vi "VLT.vi"() -> ()   [LabVIEW 2025]
uses:
  <vilib>/sound2/lvsound2.llb/Sound Data Format.ctl
  <vilib>/sound2/lvsound2.llb/Sampling Mode.ctl
  <vilib>/sound2/lvsound2.llb/Sound Input Task ID.ctl
  <vilib>/sound2/lvsound2.llb/Sound Output Task ID.ctl
  <vilib>/sound2/lvsound2.llb/Sound Output Write (DBL Single).vi
  <vilib>/sound2/lvsound2.llb/Sound Output Set Volume (Single).vi
  <vilib>/sound2/lvsound2.llb/Sound Input Read (DBL).vi
  <vilib>/Analysis/NI_AALBase.lvlib
  <vilib>/measure/NI_MABase.lvlib
  <vilib>/Utility/inputDevices.llb/joystickAcquire.vi
  <vilib>/sound2/lvsound2.llb/Sound Output Write (DBL).vi
  <vilib>/sound2/lvsound2.llb/Sound File Write Open.vi
  <vilib>/sound2/lvsound2.llb/Sound File Write (DBL).vi
panel:
  in  "Tone Volume":dbl(slide) scale=0.0..1.0 scale format="%_1f"
  out "sample rate (S/s)":dbl
  in  "Sound Waves 2":u16(ring) items=["Sine Wave", "Triangle Wave", "Sawtooth Wave"]
  out "Tone Generator 2":dbl
  out "Number of Samples/ch":i32=20000
  in  "Exit":bool
  in  "stapu 2":bool
  in  "Stop Program":bool
  in  "Input Devicea ID":dbl
  in  "Output Volume":dbl(slide) scale=0.0..100.0
  in  "Sound Devicea ID":dbl
  in  "Pause":bool
  out "Error Write":bool
  in  "Sound Format":T1={"sample rate (S/s)"=22050.0, "number of channels"=2, "bits per sample"=16}
  in  "Record Stop":bool
  out "Error Read":bool
  in  "VLT":T2(tab)
  in  "Playback":bool
  out "Pitch (Hz)":dbl format="%#.2f"
  out "Amplitude Tracker":dynamicdata(graph) caption="Frequency"
  out "Pitch Tracker":waveform(dbl)(graph) caption="Frequency"
  out "Low (Hz)":dbl format="%#.1f"
  out "High (Hz)":dbl format="%#.1f"
  out "Volume (dB)":dbl format="%#.2f"
  out "High (dB)":dbl format="%#.2f"
  out "Low (dB)":dbl format="%#.2f"
  in  "Sound Patterns":u16(ring)
  in  "Sound Waves":u16(ring) items=["Sine Wave", "Triangle Wave", "Sawtooth Wave", "Test"]
  in  "Tone Buttons":T3(radio)=enum."92"
  out "Sound Input":dbl format="%#.0f"
  out "Tone Generator":u32
  # "Hz"
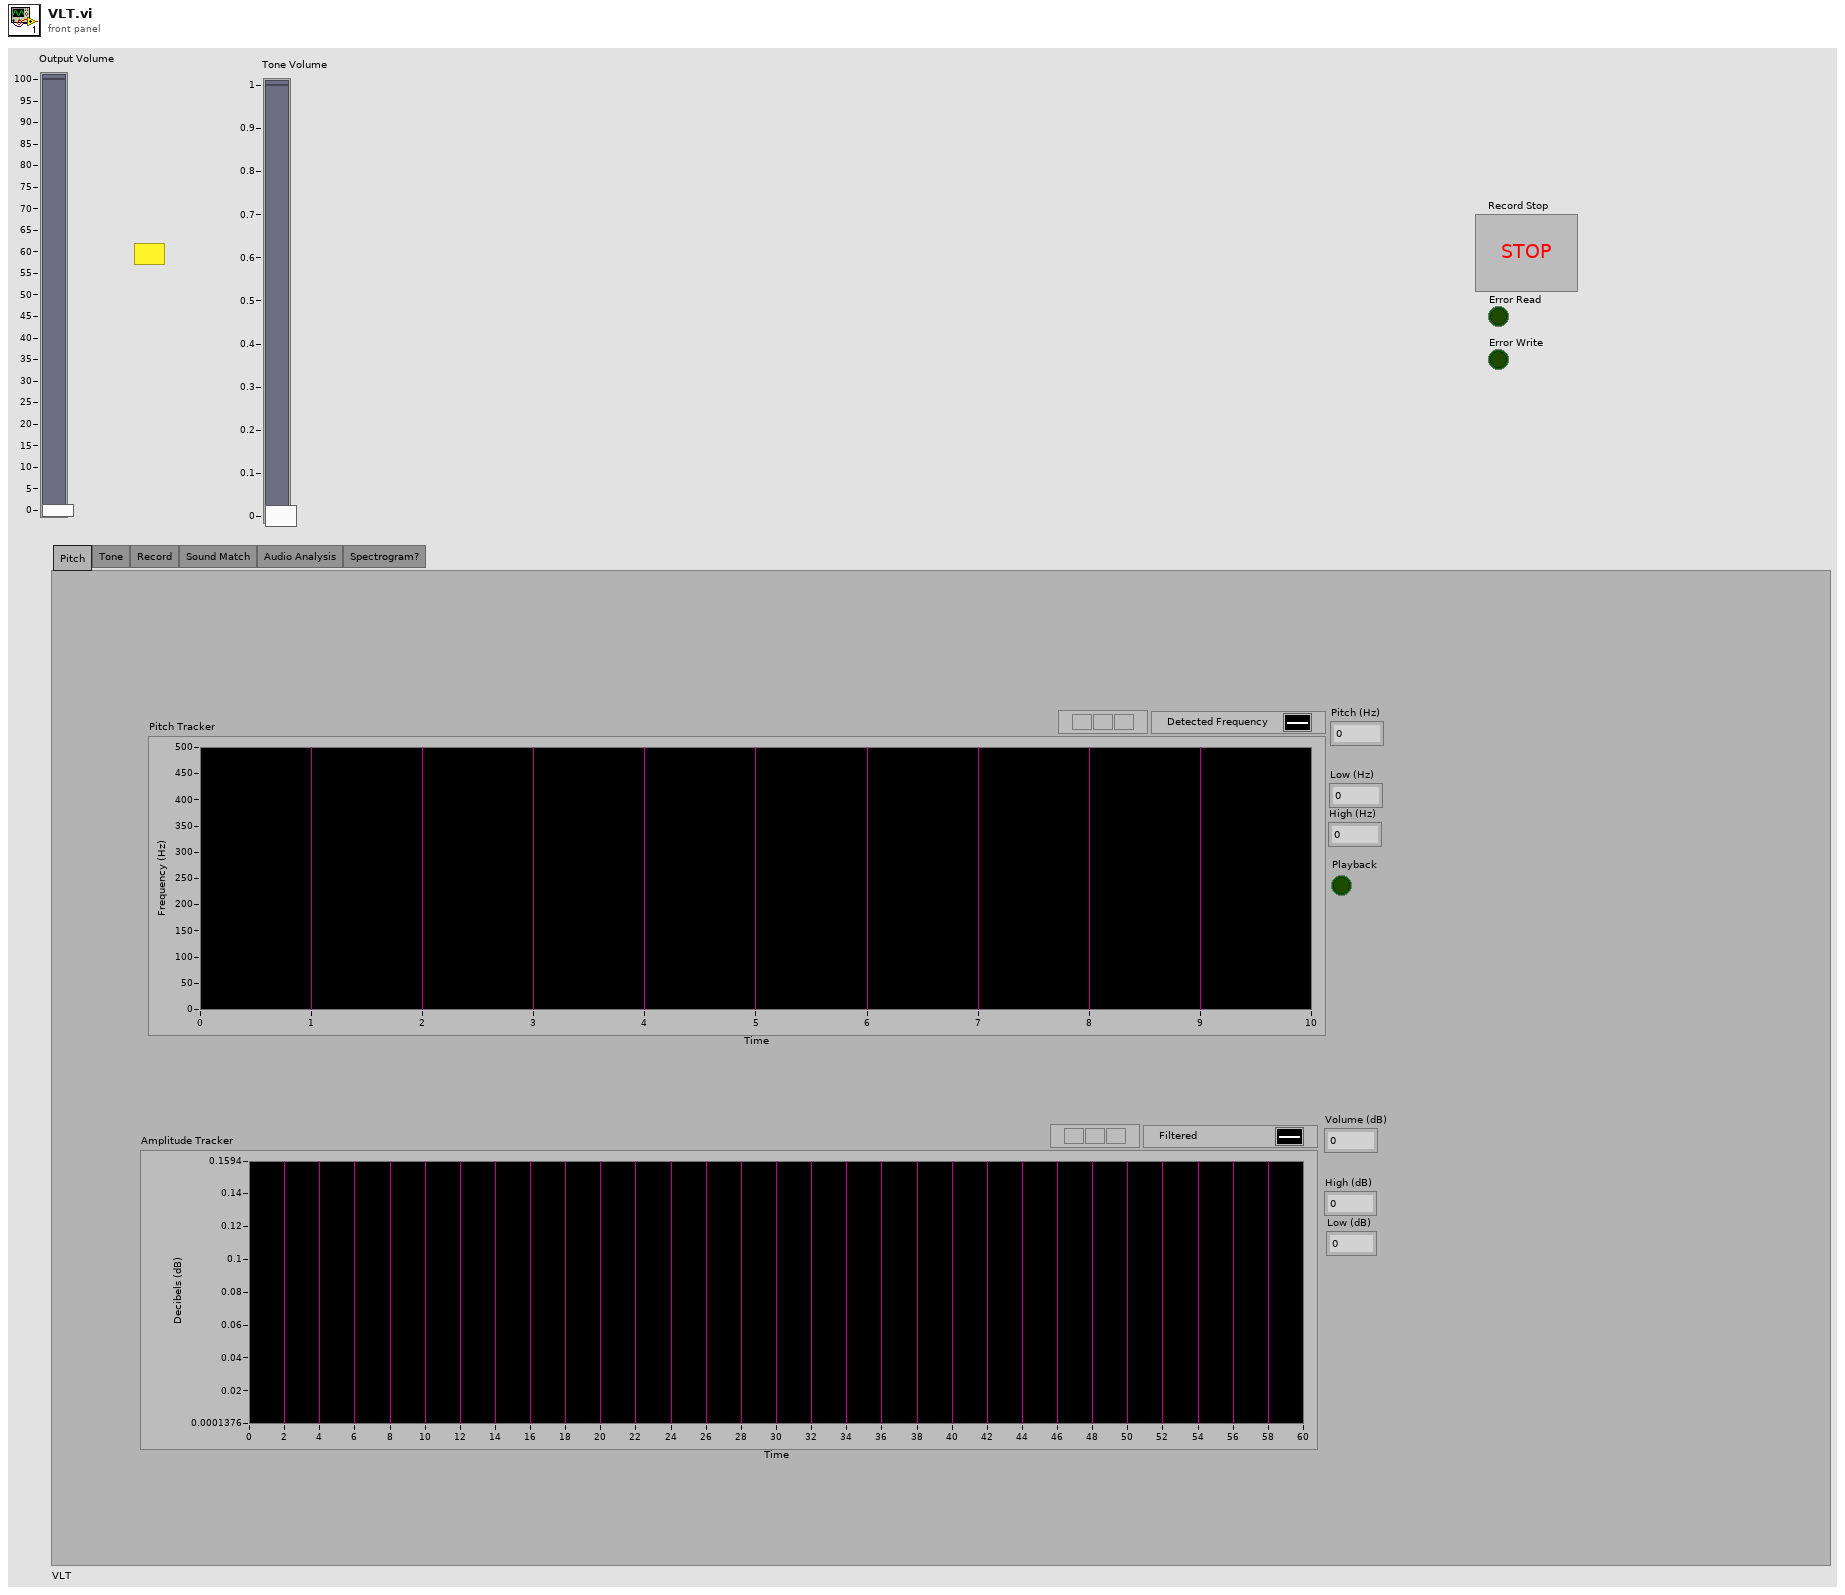
[diagram p1: front panel]
types:
  T1 = typedef "Sound Data Format.ctl" = cluster{"sample rate (S/s)":dbl, "number of channels":i32, "bits per sample":i32}
  T2 = enum32{"Pitch", "Tone", "Record", "Sound Match", "Audio Analysis", "Spectrogram?"}
  T3 = enum32{"No Selection", "92", "98", "104", "110", "117", "123", "175", "165", "156", "131", "139", "147", "247", "233", "220", "185", "196", "208", "349", "330", "311", "262", "277", "294"}
  T4 = typedef "Sound Output Task ID.ctl" = u32
  T5 = typedef "Sound Input Task ID.ctl" = u32
  T6 = typedef "Sampling Mode.ctl" = i32
  T7 = typedef "Sound File Refnum.ctl" = refnum<file>
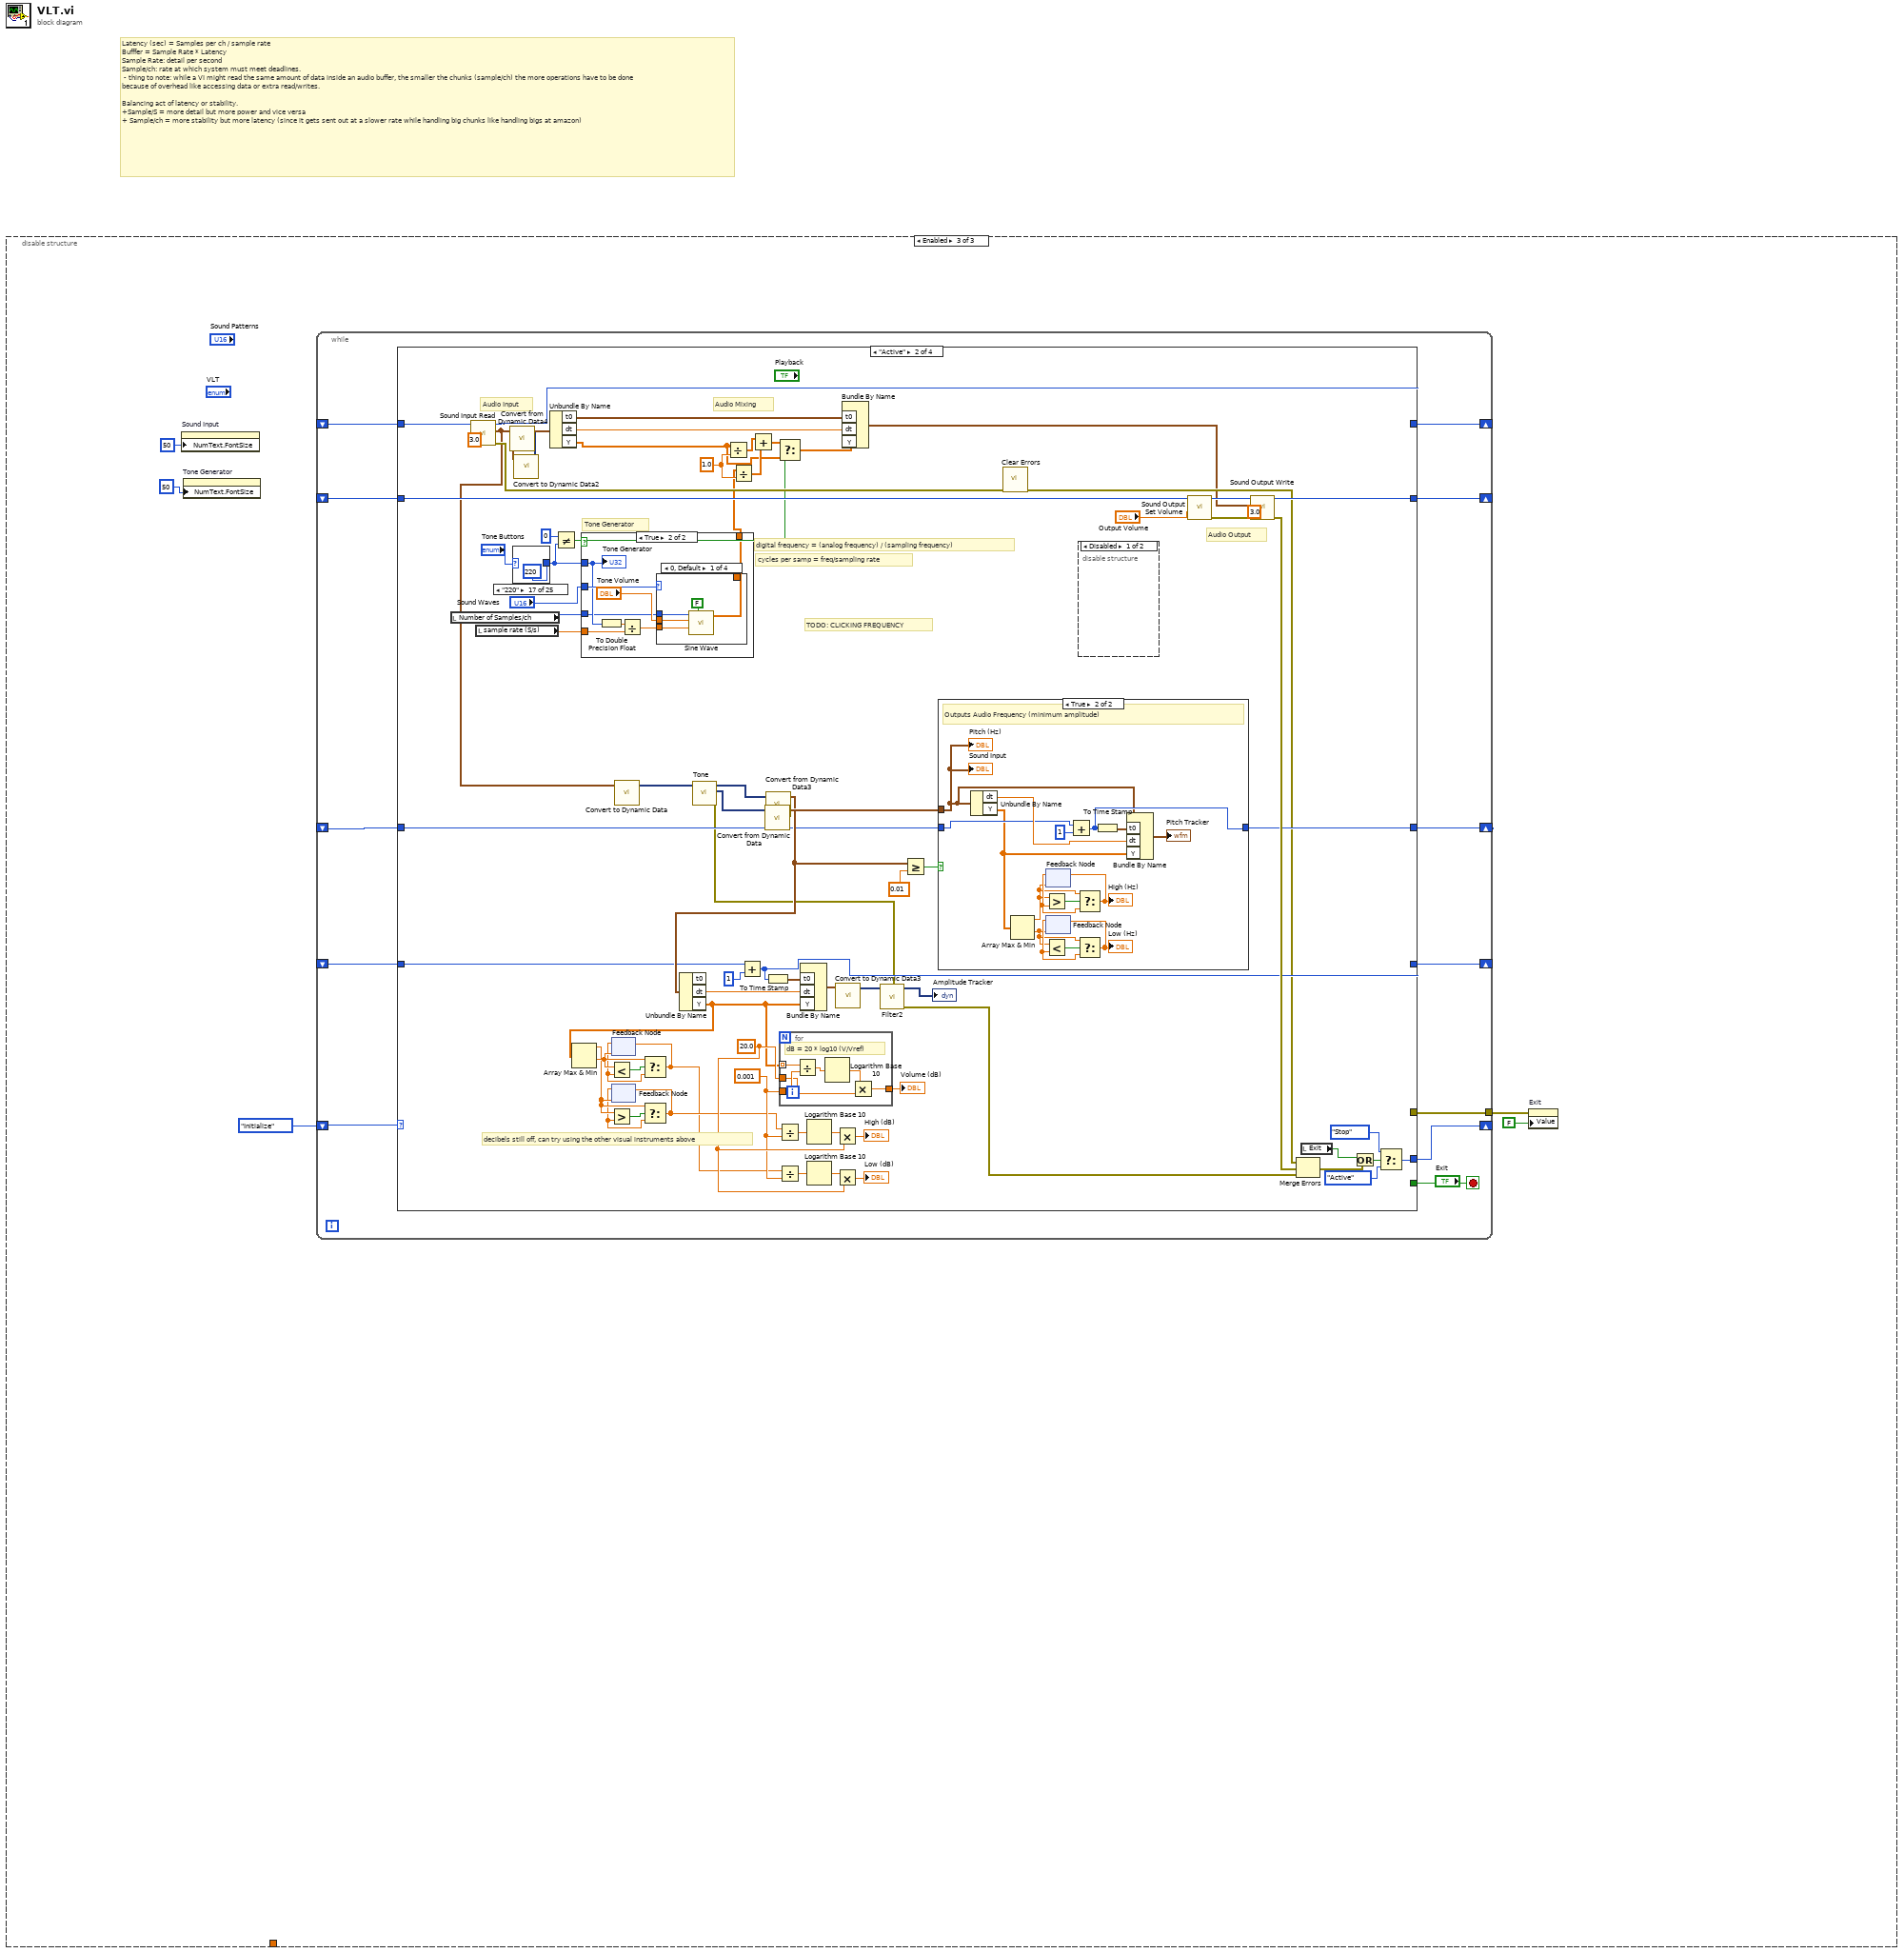
[diagram p0: block diagram]
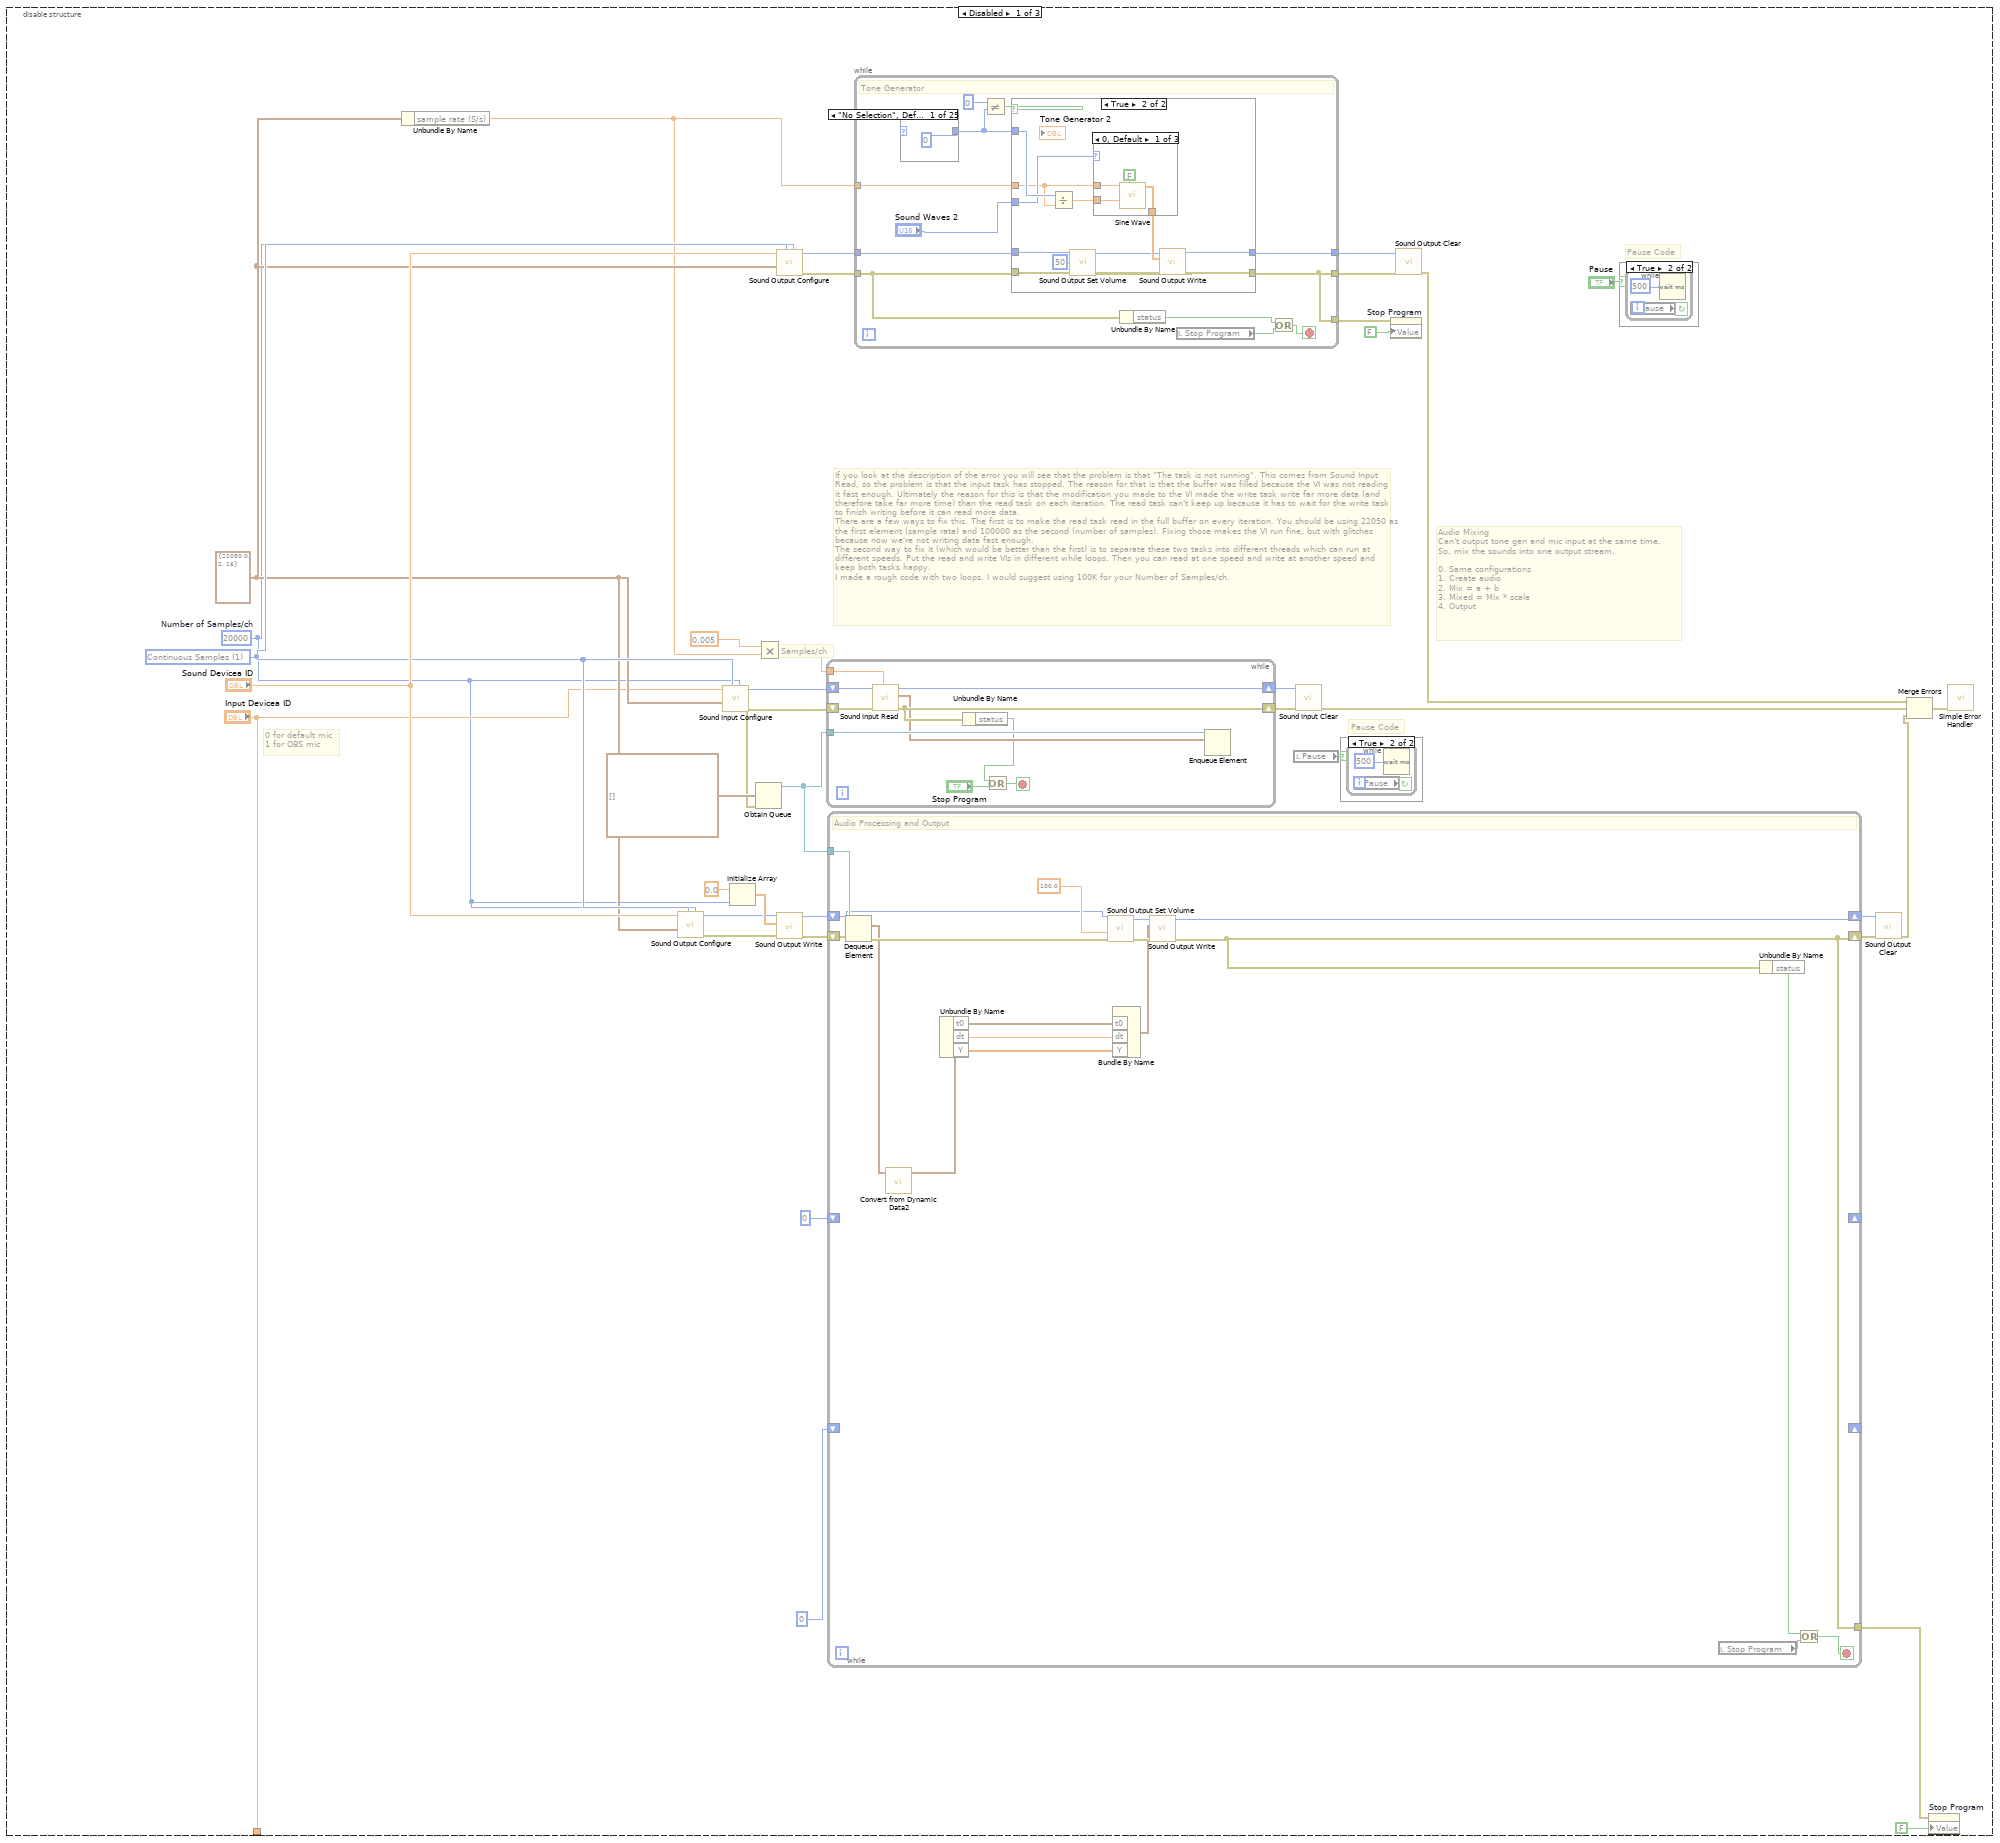
[diagram p2: hidden frame]
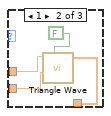
[diagram p6: hidden frame]
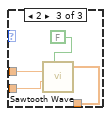
[diagram p7: hidden frame]
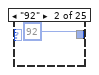
[diagram p8: hidden frame]
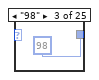
[diagram p9: hidden frame]
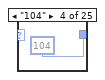
[diagram p10: hidden frame]
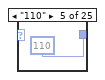
[diagram p11: hidden frame]
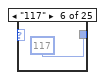
[diagram p12: hidden frame]
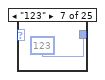
[diagram p13: hidden frame]
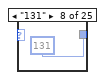
[diagram p14: hidden frame]
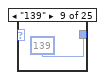
[diagram p15: hidden frame]
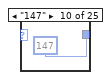
[diagram p16: hidden frame]
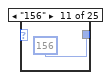
[diagram p17: hidden frame]
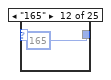
[diagram p18: hidden frame]
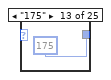
[diagram p19: hidden frame]
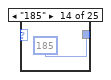
[diagram p20: hidden frame]
diagram:
  # "Latency (sec) = Samples per ch / sample rate\nBufffer = Sample Rate * Latency\nSample Rate: detail per second\nSample/ch: rate at which system must meet deadlines.\n - thing to note: while a VI might read the same amount of data inside an audio buffer, the smaller the chunks (sample/ch) the more operations have to be done because of overhead like accessing data or extra read/writes.\n\nBalancing act of latency or stability. \n+Sample/S = more detail but more power and vice versa\n+ Sample/ch = more stability but more latency (since it gets sent out at a slower rate while handling big chunks like handling bigs at amazon)"
  n1 = disable-structure shown="Enabled" {
    disable-tunnel: ["Input Devicea ID" _ _] -> _
    frame Disabled {
      w11 = T1 {"sample rate (S/s)"=22050.0, "number of channels"=2, "bits per sample"=16} ("sound format")
      w2 = 20000  # Number of Samples/ch
      w37 = T6 1 items=["Finite Samples", "Continuous Samples"] ("sample mode")
      # "Pause Code"
      # "Audio Mixing\nCan't output tone gen and mic input at the same time.\nSo, mix the sounds into one output stream.\n\n0. Same configurations\n1. Create audio\n2. Mix = a + b\n3. Mixed = Mix * scale\n4. Output"
      # "Pause Code"
      # "Samples/ch"
      # "If you look at the description of the error you will see that the problem is that \"The task is not running\". This comes from Sound Input Read, so the problem is that the input task has stopped. The reason for that is that the buffer was filled because the VI was not reading it fast enough. Ultimately the reason for this is that the modification you made to the VI made the write task write far more data (and therefore take far more time) than the read task on each iteration. The read task can't keep up because it has to wait for the write task to finish writing before it can read more data.\nThere are a few ways to fix this. The first is to make the read task read in the full buffer on every iteration. You should be using 22050 as the first element (sample rate) and 100000 as the second (number of samples). Fixing those makes the VI run fine, but with glitches because now we're not writing data fast enough.\nThe second way to fix it (which would be better than the first) is to separate these two tasks into different threads which can run at different speeds. Put the read and write VIs in different while loops. Then you can read at one speed and write at another speed and keep both tasks happy.\nI made a rough code with two loops. I would suggest using 100K for your Number of Samples/ch."
      # "0 for default mic\n1 for OBS mic"
      n2 = Unbundle By Name(w11) -> ("sample rate (S/s)"=w3:dbl)
      n3 = call <vilib>:"Sound Output Configure.vi"("number of samples/ch"=w2, "sample mode"=w37, "sound format"=w11, "device ID"="Sound Devicea ID") -> ("error out"=w26:errorcluster, "task ID"=w27:T4)  [unwired: 6 in]
      n4 = call <vilib>:"Sound Input Configure.vi"("number of samples/ch"=w2, "sample mode"=w37, "sound format"=w11, "device ID"="Input Devicea ID") -> ("error out"=w16:errorcluster, "task ID"=w19:T5)  [unwired: 6 in]
      n5 = Initialize Array(0.0 ("element"), w2) -> (w30:dbl[])
      n6 = Obtain Queue(element data type=waveform(dbl)[] [] ("data"), error in (no error)=w16) -> (queue out=w22:refnum<queue>)  [unwired: 2 in, 3 out]
      n7 = Multiply(x=0.005, y=w3) -> (x*y=w12:dbl)
      n8 = call <vilib>:"Sound Output Configure.vi"("number of samples/ch"=w2, "sample mode"=w37, "sound format"=w11, "device ID"="Sound Devicea ID") -> ("error out"=w35:errorcluster, "task ID"=w36:T4)  [unwired: 6 in]
      n9 = call-poly <vilib>:"Sound Output Write.vi"("error in (no error)"=w26, "data"=w30, "task ID"=w27) -> ("error out"=w20:errorcluster, "task ID out"=w21:T4)  [unwired: 7 in]
      n10 = while {
        tunnel: w12 -> [w65]
        tunnel: w22 -> [w64]
        shift-right: [w66] -> w18
        shift-left: w19 -> [w69]
        shift-right: [w67] -> w17
        shift-left: w16 -> [w68]
        stop <- w70 stop-if-true
        # "Audio Input Queue"
        n11 = call-poly <vilib>:"Sound Input Read.vi"("number of samples/ch"=w65, "error in (no error)"=w68, "task ID"=w69) -> ("error out"=w67:errorcluster, "data"=w63:waveform(dbl)[], "task ID out"=w66:T5)  [unwired: 1 in, 5 out]
        n12 = Unbundle By Name(w67) -> ("status"=w61:bool)
        n13 = Or(x=w61, y="Stop Program") -> (x .or. y?=w70:bool)
        n14 = Enqueue Element(queue=w64, element=w63) -> ()  [unwired: 1 in, 4 out]
      }
      n15 = while {
        shift-right: _ -> [_]
        shift-left: 0 -> [_]
        shift-right: _ -> [_]
        shift-left: 0 -> [_]
        tunnel: w22 -> [w60]
        tunnel: [w49] -> w14
        shift-right: [w53] -> w8
        shift-left: w21 -> [w51]
        shift-right: [w49] -> w9
        shift-left: w20 -> [w57]
        stop <- w59 stop-if-true
        # "Audio Processing and Output"
        n16 = Dequeue Element(queue=w60, error in (no error)=w57) -> (element=w50:waveform(dbl)[], error out=w52:errorcluster)  [unwired: 3 out]
        n17 = call "Convert from Dynamic Data2"("Dynamic Data Type"=w50) -> ("Waveform"=w43:waveform(dbl))  [unwired: 3 in]
        n18 = Unbundle By Name(w43) -> ("t0"=w44:timestamp, "dt"=w47:dbl, "Y"=w46:dbl[])
        n19 = call-poly <vilib>:"Sound Output Set Volume.vi"("error in (no error)"=w52, "volume"=100.0 ("Volume 2"), "task ID"=w51) -> ("error out"=w54:errorcluster, "task ID out"=w55:T4)  [unwired: 7 in]
        n20 = Bundle By Name("t0"=w44, "dt"=w47, "Y"=w46) -> (w45:waveform(dbl))  [unwired: 1 in]
        n21 = call-poly <vilib>:"Sound Output Write.vi"("error in (no error)"=w54, "data"=w45, "task ID"=w55) -> ("error out"=w49:errorcluster, "task ID out"=w53:T4)  [unwired: 7 in]
        n22 = local read "Stop Program"() -> (w58:bool)
        n23 = Unbundle By Name(w49) -> ("status"=w48:bool)
        n24 = Or(x=w48, y=w58) -> (x .or. y?=w59:bool)
      }
      n25 = while {
        tunnel: w3 -> [w81]
        tunnel: w36 -> [w82]
        tunnel: [w80] -> w34
        tunnel: w35 -> [w79]
        tunnel: [w72] -> w33
        tunnel: [w72] -> w6
        stop <- w75 stop-if-true
        # "Tone Generator"
        n26 = case shown="\"No Selection\", Default" {
          selector: _ -> [_ _ _ _ _ _ _ _ _ _ _ _ _ _ _ _ _ _ _ _ _ _ _ _ _]
          tunnel: [u32 0 ("Tone Buttons") u32 92 ("Tone Buttons") u32 98 ("Tone Buttons") 104 110 u32 117 ("Tone Buttons") u32 123 ("Tone Buttons") u32 131 ("Tone Buttons") u32 139 ("Tone Buttons") u32 147 ("Tone Buttons") u32 156 ("Tone Buttons") u32 165 ("Tone Buttons") u32 175 ("Tone Buttons") u32 185 ("Tone Buttons") u32 196 ("Tone Buttons") u32 208 ("Tone Buttons") u32 220 ("Tone Buttons") u32 233 ("Tone Buttons") u32 247 ("Tone Buttons") u32 262 ("Tone Buttons") u32 277 ("Tone Buttons") u32 294 ("Tone Buttons") u32 311 ("Tone Buttons") u32 330 ("Tone Buttons") u32 349 ("Tone Buttons")] -> w78
          frame "No Selection", Default {
          }
          frame "92" {
          }
          frame "98" {
          }
          frame "104" {
          }
          frame "110" {
          }
          frame "117" {
          }
          frame "123" {
          }
          frame "131" {
          }
          frame "139" {
          }
          frame "147" {
          }
          frame "156" {
          }
          frame "165" {
          }
          frame "175" {
          }
          frame "185" {
          }
          frame "196" {
          }
          frame "208" {
          }
          frame "220" {
          }
          frame "233" {
          }
          frame "247" {
          }
          frame "262" {
          }
          frame "277" {
          }
          frame "294" {
          }
          frame "311" {
          }
          frame "330" {
          }
          frame "349" {
          }
        }
        n27 = Not Equal?(x=u32 0, y=w78) -> (x != y?=w76:bool)
        n28 = case shown="True" w76 {
          tunnel: w82 -> [w84 w90]
          tunnel: w81 -> [_ w85]
          tunnel: [w83 w87] -> w72
          tunnel: [w84 w88] -> w80
          tunnel: w79 -> [w83 w92]
          tunnel: w78 -> [_ w94]
          tunnel: "Sound Waves 2" -> [_ w93]
          frame False {
          }
          frame True {
            n29 = Divide(x=w94, y=w85) -> (x/y=w96:dbl)
            n30 = call-poly <vilib>:"Sound Output Set Volume.vi"("error in (no error)"=w92, "volume"=50, "task ID"=w90) -> ("error out"=w91:errorcluster, "task ID out"=w89:T4)  [unwired: 7 in]
            n31 = case shown="0, Default" w93 {
              tunnel: w85 -> [w100 w104 w105]
              tunnel: w96 -> [w99 w103 w106]
              tunnel: [w98 w102 w107] -> w95
              frame 0, Default {
                n32 = call <vilib>:"Sine Wave.vi"("samples"=w100, "frequency"=w99, "reset phase"=FALSE) -> ("sine wave"=w98:dbl[])  [unwired: 2 in, 2 out]
              }
              frame 1 {
                n33 = call <vilib>:"Triangle Wave.vi"("samples"=w104, "frequency"=w103, "reset phase"=FALSE) -> ("triangle wave"=w102:dbl[])  [unwired: 2 in, 2 out]
              }
              frame 2 {
                n34 = call <vilib>:"Sawtooth Wave.vi"("samples"=w105, "frequency"=w106, "reset phase"=FALSE) -> ("sawtooth wave"=w107:dbl[])  [unwired: 2 in, 2 out]
              }
            }
            n35 = call-poly <vilib>:"Sound Output Write.vi"("error in (no error)"=w91, "data"=w95, "task ID"=w89) -> ("error out"=w87:errorcluster, "task ID out"=w88:T4)  [unwired: 7 in]
          }
        }
        n36 = Unbundle By Name(w79) -> ("status"=w74:bool)
        n37 = local read "Stop Program"() -> (w73:bool)
        n38 = Or(x=w74, y=w73) -> (x .or. y?=w75:bool)
      }
      n39 = local read "Pause"() -> (w4:bool)
      n40 = call <vilib>:"Sound Input Clear.vi"("error in (no error)"=w17, "task ID"=w18) -> ("error out"=w32:errorcluster)  [unwired: 9 in]
      n41 = case shown="True" w4 {
        frame False {
        }
        frame True {
          n42 = while {
            stop <- w41 continue-if-true
            n43 = local read "Pause"() -> (w41:bool)
            n44 = Wait (ms)(milliseconds to wait=u32 500) -> ()  [unwired: 1 out]
          }
        }
      }
      n45 = property on="Stop Program" class="Bool (strict)"(error in=w6, "Value"=FALSE) -> ()  [unwired: 1 in, 2 out]
      n46 = call <vilib>:"Sound Output Clear.vi"("error in (no error)"=w33, "task ID"=w34) -> ("error out"=w5:errorcluster)  [unwired: 9 in]
      n47 = case shown="True" "Pause" {
        frame False {
        }
        frame True {
          n48 = while {
            stop <- w39 continue-if-true
            n49 = local read "Pause"() -> (w39:bool)
            n50 = Wait (ms)(milliseconds to wait=u32 500) -> ()  [unwired: 1 out]
          }
        }
      }
      n51 = call <vilib>:"Sound Output Clear.vi"("error in (no error)"=w9, "task ID"=w8) -> ("error out"=w28:errorcluster)  [unwired: 9 in]
      n52 = Merge Errors(w5, w32, w28) -> (w31:errorcluster)
      n53 = property on="Stop Program" class="Bool (strict)"(error in=w14, "Value"=FALSE) -> ()  [unwired: 1 in, 2 out]
      n54 = call <vilib>:"Simple Error Handler.vi"("error in (no error)"=w31) -> ()  [unwired: 4 in, 5 out]
    }
    frame Disabled {
      w155 = T6 1 items=["Finite Samples", "Continuous Samples"] ("sample mode")
      w164 = 20000  # Number of Samples/ch
      w177 = T1 {"sample rate (S/s)"=88200.0, "number of channels"=2, "bits per sample"=16} ("Sound Format")
      w180 = T6 1 items=["Finite Samples", "Continuous Samples"] ("sample mode")
      # "audio recording test"
      # "+quality < -quality\n-speed < +speed"
      # "Audio input testing with waveform fed into a queue and outputted in another while loop"
      n55 = call <vilib>:"Dflt Data Dir.vi"() -> ()  [unwired: 1 out]
      n56 = call "File Dialog2"("default name"="test.wav", "pattern (all files)"="*.wav" ("DNL_pattern"), "pattern label"="Sound files") -> ("selected path"=w150:path, "error out"=w158:errorcluster)  [unwired: 4 in, 7 out]
      n57 = Unbundle By Name("Sound Format") -> ("sample rate (S/s)"=w149:dbl)
      n58 = call <vilib>:"Sound Output Configure.vi"("number of samples/ch"=w164, "sample mode"=w180, "sound format"=w177, "device ID"=0) -> ("error out"=w178:errorcluster, "task ID"=w179:T4)  [unwired: 6 in]
      n59 = Initialize Array(0.0 ("element"), w164) -> (w175:dbl[])
      n60 = call-poly <vilib>:"Sound Output Write.vi"("error in (no error)"=w178, "data"=w175, "task ID"=w179) -> ("error out"=w168:errorcluster, "task ID out"=w169:T4)  [unwired: 7 in]
      n61 = call <vilib>:"Sound Input Configure.vi"("number of samples/ch"=w164, "sample mode"=w180, "sound format"=w177, "device ID"=1) -> ("error out"=w167:errorcluster, "task ID"=w173:T5)  [unwired: 6 in]
      n62 = Obtain Queue(element data type=waveform(dbl)[] [] ("data"), error in (no error)=w167) -> (queue out=w170:refnum<queue>)  [unwired: 2 in, 3 out]
      n63 = Quotient & Remainder(x=w164, y=2) -> (floor(x/y)=w172:i32)  [unwired: 1 out]
      n64 = Divide(x=w149, y=12.0) -> (x/y=w147:dbl)
      n65 = while {
        tunnel: [w212] -> w162
        tunnel: [w205] -> w161
        tunnel: w170 -> [w211]
        tunnel: w169 -> [w209]
        tunnel: w168 -> [w208]
        tunnel: [w205] -> w166
        stop <- w206 stop-if-true
        n66 = Dequeue Element(queue=w211, error in (no error)=w208) -> (element=w210:waveform(dbl)[], error out=w207:errorcluster)  [unwired: 3 out]
        n67 = local read "stapu 2"() -> (w206:bool)
        n68 = call-poly <vilib>:"Sound Output Write.vi"("error in (no error)"=w207, "data"=w210, "task ID"=w209) -> ("error out"=w205:errorcluster, "task ID out"=w212:T4)  [unwired: 7 in]
      }
      n69 = while {
        tunnel: w172 -> [_]
        tunnel: w173 -> [w220]
        tunnel: [w219] -> w182
        tunnel: w167 -> [w218]
        tunnel: [w216] -> w181
        tunnel: w170 -> [w215]
        tunnel: 220 ("Number of Samples/ch") -> [w213]
        stop <- "stapu 2" stop-if-true
        # "Proper Sound Playback"
        n70 = call-poly <vilib>:"Sound Input Read.vi"("number of samples/ch"=w213, "error in (no error)"=w218, "task ID"=w220) -> ("error out"=w216:errorcluster, "data"=w214:waveform(dbl)[], "task ID out"=w219:T5)  [unwired: 6 in]
        n71 = Enqueue Element(queue=w215, element=w214) -> ()  [unwired: 1 in, 4 out]
      }
      n72 = To Long Integer(number=w147) -> (32bit integer=w145:i32)
      n73 = call-poly <vilib>:"Sound File Open.vi"("error in (no error)"=w158, "sound format"="Sound Format", "path"=w150) -> ("error out"=w157:errorcluster, "sound file refnum"=w156:T7)  [unwired: 7 out]
      n74 = call <vilib>:"Sound Input Clear.vi"("error in (no error)"=w181, "task ID"=w182) -> ()  [unwired: 9 in, 1 out]
      n75 = property on="stapu 2" class="Bool (strict)"(error in=w166, "Value"=FALSE) -> ()  [unwired: 1 in, 2 out]
      n76 = call <vilib>:"Sound Input Configure.vi"("number of samples/ch"=w145, "sample mode"=w155, "error in (no error)"=w157, "sound format"="Sound Format") -> ("error out"=w135:errorcluster, "task ID"=w154:T5, "device ID"=w134:u32)  [unwired: 1 in, 4 out]
      n77 = call <vilib>:"Sound Output Clear.vi"("error in (no error)"=w161, "task ID"=w162) -> ()  [unwired: 9 in, 1 out]
      n78 = Obtain Queue(element data type=waveform(dbl)[] [] ("data"), error in (no error)=w135) -> (queue out=w137:refnum<queue>)  [unwired: 2 in, 3 out]
      n79 = call "File Dialog"() -> ()  [unwired: 12 in, 4 out]
      n80 = call-poly <vilib>:"Acquire Input Data.vi"() -> ()  [unwired: 15 in, 5 out]
      n81 = call "Filter"() -> ()  [unwired: 10 in, 2 out]
      n82 = call "Select Signals"() -> ()  [unwired: 10 in, 2 out]
      n83 = call "Amplitude and Level Measurements"() -> ()  [unwired: 8 in, 8 out]
      n84 = while {
        tunnel: w145 -> [w201]
        shift-right: [w202] -> w139
        shift-left: w154 -> [w203]
        shift-right: [w194] -> w138
        shift-left: w135 -> [w204]
        tunnel: w137 -> [w195]
        stop <- w198 stop-if-true
        # "3."
        n85 = call-poly <vilib>:"Sound Input Read.vi"("number of samples/ch"=w201, "error in (no error)"=w204, "task ID"=w203) -> ("error out"=w197:errorcluster, "data"=w196:waveform(dbl)[], "task ID out"=w202:T5)  [unwired: 1 in, 5 out]
        n86 = Enqueue Element(queue=w195, element=w196, error in (no error)=w197) -> (error out=w194:errorcluster)  [unwired: 3 out]
        n87 = Unbundle By Name(w194) -> ("status"=w200:bool)
        "Error Read" <- w200
        n88 = Or(x=w200, y="Record Stop") -> (x .or. y?=w198:bool)
        n89 = Wait (ms)(milliseconds to wait=u32 20) -> ()  [unwired: 1 out]
      }
      n90 = while {
        tunnel: w135 -> [w190]
        tunnel: w137 -> [w191]
        shift-right: [w188] -> w142
        shift-left: w156 -> [w192]
        tunnel: [w183] -> w141
        stop <- w185 stop-if-true
        n91 = Dequeue Element(queue=w191, error in (no error)=w190) -> (element=w187:waveform(dbl)[], error out=w189:errorcluster)  [unwired: 3 out]
        n92 = call-poly <vilib>:"Sound File Write.vi"("error in (no error)"=w189, "data"=w187, "sound file refnum"=w192) -> ("error out"=w183:errorcluster, "sound file refnum out"=w188:T7)  [unwired: 7 out]
        n93 = local read "Record Stop"() -> (w186:bool)
        n94 = Unbundle By Name(w183) -> ("status"=w184:bool)
        "Error Write" <- w184
        n95 = Or(x=w184, y=w186) -> (x .or. y?=w185:bool)
      }
      n96 = call "Align and Resample"() -> ()  [unwired: 9 in, 3 out]
      n97 = call "Elapsed Time"() -> ()  [unwired: 12 in, 8 out]
      n98 = call "Distortion Measurements"() -> ()  [unwired: 8 in, 4 out]
      n99 = property on="Record Stop" class="Bool (strict)"(error in=w141, "Value"=FALSE ("stop")) -> ()  [unwired: 1 in, 2 out]
      n100 = call <vilib>:"Sound Input Clear.vi"("error in (no error)"=w138, "task ID"=w139) -> ("error out"=w143:errorcluster)  [unwired: 9 out]
      n101 = call <vilib>:"Sound File Close.vi"("error in (no error)"=w143, "sound file refnum"=w142) -> ("error out"=w144:errorcluster)  [unwired: 9 out]
      n102 = call <vilib>:"Simple Error Handler.vi"("error in (no error)"=w144) -> ()  [unwired: 1 in, 8 out]
    }
    frame Enabled {
      n103 = property on="Sound Input" class="DigNum (strict)"("NumText.FontSize"=u32 50 ("Numeric Text.Font:Size")) -> ()  [unwired: 2 in, 2 out]
      n104 = property on="Tone Generator" class="DigNum (strict)"("NumText.FontSize"=u32 50 ("Numeric Text.Font:Size")) -> ()  [unwired: 2 in, 2 out]
      n105 = while {
        shift-right: [w235] -> _
        shift-left: _ -> [w231]
        shift-right: [w236] -> _
        shift-left: _ -> [w232]
        shift-right: [w234] -> _
        shift-left: enum16{"Initialize", "Active", "Stop", "Exit"}."Initialize" -> [w237]
        tunnel: [w230] -> w223
        shift-right: [w228] -> _
        shift-left: _ -> [w229]
        shift-right: [w226] -> _
        shift-left: _ -> [w227]
        stop <- w233 stop-if-true
        n106 = case shown="\"Active\"" w237 {
          tunnel: [w258 w337 T5 0 ("task ID out") T5 0 ("task ID out")] -> w236
          tunnel: [w246 w336 T4 0 ("task ID out") T4 0 ("task ID out")] -> w235
          tunnel: [w255 w333 w415 w437] -> w234
          tunnel: [_ _ _ TRUE] -> w233
          tunnel: w232 -> [_ w338 w420 w439]
          tunnel: w231 -> [_ w286 w419 w438]
          tunnel: [_ _ _ w433] -> w230
          tunnel: w229 -> [_ w293 _ _]
          tunnel: [_ w292 _ 0] -> w228
          tunnel: w227 -> [_ w291 _ _]
          tunnel: [_ w290 _ 0] -> w226
          frame "Initialize" {
            w242 = u32 0  # Input Device ID
            w243 = u32 0  # Sound Device ID
            w244 = T1 {"sample rate (S/s)"=88200.0, "number of channels"=2, "bits per sample"=16} ("sound format")
            (unwired) 20000  # Number of Samples/ch
            w263 = T6 1 items=["Finite Samples", "Continuous Samples"] ("sample mode")
            n107 = Unbundle By Name(w244) -> ("sample rate (S/s)"=w240:dbl)
            "sample rate (S/s)" <- w240
            n108 = Divide(x=w240, y=4.0) -> (x/y=w241:dbl)
            n109 = To Long Integer(number=w241) -> (32bit integer=w239:i32)
            "Number of Samples/ch" <- w239
            n110 = call <vilib>:"Sound Output Configure.vi"("number of samples/ch"=w239, "sample mode"=w263, "sound format"=w244, "device ID"=w243) -> ("error out"=w259:errorcluster, "task ID"=w260:T4)  [unwired: 6 in]
            n111 = call <vilib>:"Sound Input Configure.vi"("number of samples/ch"=w239, "sample mode"=w263, "sound format"=w244, "device ID"=w242) -> ("error out"=w261:errorcluster, "task ID"=w262:T5)  [unwired: 6 in]
            n112 = call <vilib>:"Sound Input Start.vi"("error in (no error)"=w261, "task ID"=w262) -> ("error out"=w257:errorcluster, "task ID out"=w258:T5)  [unwired: 8 in]
            n113 = call <vilib>:"Sound Output Start.vi"("error in (no error)"=w259, "task ID"=w260) -> ("error out"=w248:errorcluster, "task ID out"=w249:T4)  [unwired: 8 in]
            n114 = Initialize Array(0.0 ("element"), w239) -> (w245:dbl[])
            n115 = call-poly <vilib>:"Sound Output Write.vi"("error in (no error)"=w248, "data"=w245, "task ID"=w249) -> ("error out"=w247:errorcluster, "task ID out"=w246:T4)  [unwired: 7 in]
            n116 = local read "Exit"() -> (w252:bool)
            n117 = Merge Errors(w257, w247) -> (w253:errorcluster)
            n118 = Or(x=w252, y=w253) -> (x .or. y?=w251:bool)
            n119 = Select(t=enum16{"Initialize", "Active", "Stop", "Exit"}."Stop", s=w251, f=enum16{"Initialize", "Active", "Stop", "Exit"}."Active") -> (s? t:f=w255:enum16{"Initialize", "Active", "Stop", "Exit"})
          }
          frame "Active" {
            w273 = 1.0 ("y")
            w315 = 0.001
            w316 = 20.0
            # "decibels still off, can try using the other visual instruments above"
            # "TODO: CLICKING FREQUENCY"
            # "cycles per samp = freq/sampling rate"
            # "digital frequency = (analog frequency) / (sampling frequency)"
            # "Tone Generator"
            # "Audio Input"
            # "Audio Output"
            # "Audio Mixing"
            n120 = local read "Number of Samples/ch"() -> (w274:i32)
            n121 = call-poly <vilib>:"Sound Input Read.vi"("timeout (sec)"=3.0, "task ID"=w338) -> ("error out"=w279:errorcluster, "data"=w266:waveform(dbl)[], "task ID out"=w337:T5)  [unwired: 2 in, 5 out]
            n122 = local read "sample rate (S/s)"() -> (w275:dbl)
            n123 = case shown="\"220\"" "Tone Buttons" {
              tunnel: [u32 0 ("Tone Buttons") u32 92 ("Tone Buttons") u32 98 ("Tone Buttons") 104 110 u32 117 ("Tone Buttons") u32 123 ("Tone Buttons") u32 131 ("Tone Buttons") u32 139 ("Tone Buttons") u32 147 ("Tone Buttons") u32 156 ("Tone Buttons") u32 165 ("Tone Buttons") u32 175 ("Tone Buttons") u32 185 ("Tone Buttons") u32 196 ("Tone Buttons") u32 208 ("Tone Buttons") u32 220 ("Tone Buttons") u32 233 ("Tone Buttons") u32 247 ("Tone Buttons") u32 262 ("Tone Buttons") u32 277 ("Tone Buttons") u32 294 ("Tone Buttons") u32 311 ("Tone Buttons") u32 330 ("Tone Buttons") u32 349 ("Tone Buttons")] -> w326
              frame "No Selection", Default {
              }
              frame "92" {
              }
              frame "98" {
              }
              frame "104" {
              }
              frame "110" {
              }
              frame "117" {
              }
              frame "123" {
              }
              frame "131" {
              }
              frame "139" {
              }
              frame "147" {
              }
              frame "156" {
              }
              frame "165" {
              }
              frame "175" {
              }
              frame "185" {
              }
              frame "196" {
              }
              frame "208" {
              }
              frame "220" {
              }
              frame "233" {
              }
              frame "247" {
              }
              frame "262" {
              }
              frame "277" {
              }
              frame "294" {
              }
              frame "311" {
              }
              frame "330" {
              }
              frame "349" {
              }
            }
            n124 = call "Convert to Dynamic Data2"("Array of Waveforms"=w266) -> ("Dynamic Data Type"=w276:dynamicdata)  [unwired: 3 in]
            n125 = call "Convert from Dynamic Data4"("Dynamic Data Type"=w276) -> ("Waveform"=w277:waveform(dbl))  [unwired: 3 in]
            n126 = Unbundle By Name(w277) -> ("t0"=w323:timestamp, "dt"=w324:dbl, "Y"=w268:dbl[])
            n127 = Not Equal?(x=u32 0, y=w326) -> (x != y?=w269:bool)
            n128 = case shown="True" w269 {
              tunnel: w274 -> [_ w363]
              tunnel: w326 -> [_ w366]
              tunnel: "Sound Waves" -> [_ w369]
              tunnel: [_ w368] -> w265
              tunnel: w275 -> [_ w362]
              frame False {
              }
              frame True {
                n129 = To Double Precision Float(number=w366) -> (double precision float=w365:dbl)
                n130 = Divide(x=w365, y=w362) -> (x/y=w364:dbl)
                n131 = case shown="0, Default" w369 {
                  tunnel: w363 -> [w374 w379 w381 _]
                  tunnel: w364 -> [w370 w378 w382 w385]
                  tunnel: [w373 w377 w383 _] -> w368
                  tunnel: "Tone Volume" -> [w371 w375 w380 w386]
                  frame 0, Default {
                    n132 = call <vilib>:"Sine Wave.vi"("samples"=w374, "amplitude"=w371, "frequency"=w370, "reset phase"=FALSE) -> ("sine wave"=w373:dbl[])  [unwired: 1 in, 2 out]
                  }
                  frame 1 {
                    n133 = call <vilib>:"Triangle Wave.vi"("samples"=w379, "amplitude"=w375, "frequency"=w378, "reset phase"=FALSE) -> ("triangle wave"=w377:dbl[])  [unwired: 1 in, 2 out]
                  }
                  frame 2 {
                    n134 = call <vilib>:"Sawtooth Wave.vi"("samples"=w381, "amplitude"=w380, "frequency"=w382, "reset phase"=FALSE) -> ("sawtooth wave"=w383:dbl[])  [unwired: 1 in, 2 out]
                  }
                  frame 3 {
                    n135 = call <vilib>:"Sine Waveform.vi"("reset signal"=FALSE, "amplitude"=w386, "frequency"=w385) -> ()  [unwired: 7 in, 2 out]
                  }
                }
                "Tone Generator" <- w366
              }
            }
            n136 = call "Convert to Dynamic Data"("Array of Waveforms"=w266) -> ("Dynamic Data Type"=w289:dynamicdata)  [unwired: 3 in]
            n137 = call "Tone"("Signals"=w289) -> ("error out"=w283:errorcluster, "Frequency"=w319:dynamicdata, "Amplitude"=w296:dynamicdata)  [unwired: 8 in]
            n138 = Divide(x=w268, y=w273) -> (x/y=w272:dbl[])
            n139 = Divide(x=w265, y=w273) -> (x/y=w271:dbl[])
            n140 = Add(x=w291, y=1) -> (x+y=w290:i32)
            n141 = Add(x=w272, y=w271) -> (x+y=w270:dbl[])
            n142 = call "Convert from Dynamic Data"("Dynamic Data Type"=w319) -> ("Waveform"=w318:waveform(dbl))  [unwired: 3 in]
            n143 = call "Convert from Dynamic Data3"("Dynamic Data Type"=w296) -> ("Waveform"=w303:waveform(dbl))  [unwired: 3 in]
            n144 = Unbundle By Name(w303) -> ("dt"=w297:dbl, "Y"=w304:dbl[])  [unwired: 1 out]
            n145 = Array Max & Min(array=w304) -> (max value=w310:dbl, min value=w311:dbl)  [unwired: 2 out]
            n146 = feedback #1(w311) -> (w302:dbl)
            n147 = Less?(x=w311, y=w302) -> (x < y?=w301:bool)
            n148 = feedback #2(w310) -> (w300:dbl)
            n149 = Greater?(x=w310, y=w300) -> (0:w299:bool)
            n150 = Select(t=w311, s=w301, f=w302) -> (s? t:f=w309:dbl)
            n151 = feedback-in #1(w309) -> ()
            n152 = Select(t=w310, s=w299, f=w300) -> (s? t:f=w314:dbl)
            n153 = feedback-in #2(w314) -> ()
            n154 = To Time Stamp(1:w290) -> (0:w298:timestamp)
            n155 = Select(t=w270, s=w269, f=w268) -> (s? t:f=w267:dbl[])
            n156 = Divide(x=w314, y=w315) -> (x/y=w312:dbl)
            n157 = Divide(x=w309, y=w315) -> (x/y=w307:dbl)
            n158 = for {
              tunnel: w304 -> [w344] mode=indexing
              tunnel: w315 -> [w340]
              tunnel: w316 -> [w339]
              tunnel: [w341] -> w305
              # "dB = 20 * log10 (V/Vref)"
              n159 = Divide(x=w344, y=w340) -> (x/y=w343:dbl)
              n160 = Logarithm Base 10(1:w343) -> (0:w342:dbl)
              n161 = Multiply(x=w342, y=w339) -> (x*y=w341:dbl)
            }
            "Volume (dB)" <- w305
            n162 = Bundle By Name("t0"=w298, "dt"=w297, "Y"=w304) -> (w281:waveform(dbl))  [unwired: 1 in]
            n163 = Logarithm Base 10(1:w312) -> (0:w313:dbl)
            n164 = Logarithm Base 10(1:w307) -> (0:w306:dbl)
            n165 = Multiply(x=w313, y=w316) -> (x*y=→"High (dB)":dbl)
            n166 = Multiply(x=w306, y=w316) -> (x*y=→"Low (dB)":dbl)
            n167 = call "Convert to Dynamic Data3"("Waveform"=w281) -> ("Dynamic Data Type"=w280:dynamicdata)  [unwired: 3 in]
            n168 = Bundle By Name("t0"=w323, "dt"=w324, "Y"=w267) -> (w264:waveform(dbl))  [unwired: 1 in]
            n169 = call "Filter2"("error in (no error)"=w283, "Signal"=w280) -> ("error out"=w282:errorcluster, "Filtered Signal"=→"Amplitude Tracker":dynamicdata)  [unwired: 8 in]
            n170 = Greater Or Equal?(x=w303, y=0.01) -> (x >= y?=w320:bool)
            n171 = case shown="True" w320 {
              tunnel: w318 -> [_ w347]
              tunnel: [w345 w359] -> w292
              tunnel: w293 -> [w345 w358]
              frame False {
              }
              frame True {
                # "Outputs Audio Frequency (minimum amplitude)"
                n172 = Unbundle By Name(w347) -> ("dt"=w360:dbl, "Y"=w348:dbl[])
                n173 = Array Max & Min(array=w348) -> (max value=w349:dbl, min value=w350:dbl)  [unwired: 2 out]
                n174 = feedback #3(w349) -> (w355:dbl)
                n175 = Greater?(x=w349, y=w355) -> (0:w356:bool)
                n176 = feedback #4(w350) -> (w352:dbl)
                n177 = Less?(x=w350, y=w352) -> (x < y?=w353:bool)
                n178 = Add(x=w358, y=1) -> (x+y=w359:i32)
                n179 = Select(t=w349, s=w356, f=w355) -> (s? t:f=w354:dbl)
                "High (Hz)" <- w354
                n180 = feedback-in #3(w354) -> ()
                n181 = Select(t=w350, s=w353, f=w352) -> (s? t:f=w351:dbl)
                "Low (Hz)" <- w351
                n182 = feedback-in #4(w351) -> ()
                n183 = To Time Stamp(1:w359) -> (0:w361:timestamp)
                n184 = Bundle By Name(cluster=w347, "t0"=w361, "dt"=w360, "Y"=w348) -> (→"Pitch Tracker":waveform(dbl))
                "Sound Input" <- w347
                "Pitch (Hz)" <- w347
              }
            }
            n185 = call <vilib>:"Clear Errors.vi"("error in (no error)"=w279) -> ("error out"=w278:errorcluster)  [unwired: 5 in, 1 out]
            n186 = disable-structure shown="Disabled" {
              frame Disabled {
              }
              frame Enabled {
              }
            }
            n187 = call-poly <vilib>:"Sound Output Set Volume.vi"("volume"="Output Volume", "task ID"=w286) -> ("error out"=w288:errorcluster, "task ID out"=w287:T4)  [unwired: 8 in]
            n188 = call-poly <vilib>:"Sound Output Write.vi"("timeout (sec)"=3.0, "error in (no error)"=w288, "data"=w264, "task ID"=w287) -> ("error out"=w328:errorcluster, "task ID out"=w336:T4)  [unwired: 6 in]
            n189 = Merge Errors(w278, w328, w282) -> (w327:errorcluster)
            n190 = local read "Exit"() -> (w331:bool)
            n191 = Or(x=w331, y=w327) -> (x .or. y?=w332:bool)
            n192 = Select(t=enum16{"Initialize", "Active", "Stop", "Exit"}."Stop", s=w332, f=enum16{"Initialize", "Active", "Stop", "Exit"}."Active") -> (s? t:f=w333:enum16{"Initialize", "Active", "Stop", "Exit"})
          }
          frame "Stop" {
            n193 = call <vilib>:"Sound Input Stop.vi"("task ID"=w420) -> ("error out"=w429:errorcluster, "task ID out"=w430:T5)  [unwired: 9 in]
            n194 = call <vilib>:"Sound Output Stop.vi"("task ID"=w419) -> ("error out"=w427:errorcluster, "task ID out"=w428:T4)  [unwired: 9 in]
            n195 = call <vilib>:"Sound Input Clear.vi"("error in (no error)"=w429, "task ID"=w430) -> ("error out"=w425:errorcluster)  [unwired: 9 in]
            n196 = call <vilib>:"Sound Output Clear.vi"("error in (no error)"=w427, "task ID"=w428) -> ("error out"=w426:errorcluster)  [unwired: 9 in]
            n197 = Merge Errors(w425, w426) -> (w424:errorcluster)
            n198 = call <vilib>:"Clear Errors.vi"("error in (no error)"=w424) -> ("error out"=w423:errorcluster)  [unwired: 5 in, 1 out]
            n199 = Select(t=enum16{"Initialize", "Active", "Stop", "Exit"}."Exit", s=w423, f=enum16{"Initialize", "Active", "Stop", "Exit"}."Initialize") -> (s? t:f=w416:enum16{"Initialize", "Active", "Stop", "Exit"})
            n200 = local read "Exit"() -> (w413:bool)
            n201 = Select(t=enum16{"Initialize", "Active", "Stop", "Exit"}."Exit", s=w413, f=w416) -> (s? t:f=w415:enum16{"Initialize", "Active", "Stop", "Exit"})
          }
          frame "Exit", Default {
            n202 = call <vilib>:"Sound Input Stop.vi"("task ID"=w439) -> ("error out"=w447:errorcluster, "task ID out"=w448:T5)  [unwired: 9 in]
            n203 = call <vilib>:"Sound Output Stop.vi"("task ID"=w438) -> ("error out"=w445:errorcluster, "task ID out"=w446:T4)  [unwired: 9 in]
            n204 = call <vilib>:"Sound Input Clear.vi"("error in (no error)"=w447, "task ID"=w448) -> ("error out"=w443:errorcluster)  [unwired: 9 in]
            n205 = call <vilib>:"Sound Output Clear.vi"("error in (no error)"=w445, "task ID"=w446) -> ("error out"=w444:errorcluster)  [unwired: 9 in]
            n206 = Merge Errors(w443, w444) -> (w442:errorcluster)
            n207 = call <vilib>:"Clear Errors.vi"("error in (no error)"=w442) -> ("error out"=w433:errorcluster)  [unwired: 5 in, 1 out]
            n208 = Select(t=enum16{"Initialize", "Active", "Stop", "Exit"}."Exit", s=w433, f=enum16{"Initialize", "Active", "Stop", "Exit"}."Exit") -> (s? t:f=w437:enum16{"Initialize", "Active", "Stop", "Exit"})
          }
        }
      }
      n209 = property on="Exit" class="Bool (strict)"(error in=w223, "Value"=FALSE) -> ()  [unwired: 1 in, 2 out]
    }
  }
